vi "Import Configuration and Payload Files.vi"(8 "error in":errorcluster, 9 "payload file path":path, 10 "parameters configuration file path":path, 11 "custom device ref":T1=18446744073709551615 format="%.0x") -> (0 "error out":errorcluster, 3 "custom device ref out":T1=18446744073709551615 format="%.0x")   [LabVIEW 2020, in "AIM ARINC 664 Scripting.lvlib"]
doc: "For the specified <b>custom device ref</b>, imports the parameters configuration file located at the input <b>parameters configuration file path</b>. For successful deployment and operation, the parameters configuration must be consistent with the published schema."
uses:
  AIM ARINC 664 Scripting.lvlib
  <vilib>/NI VeriStand/Custom Device API/Custom Device Item Ref.ctl
  <vilib>/NI VeriStand/Custom Device API/Custom Device API.lvlib
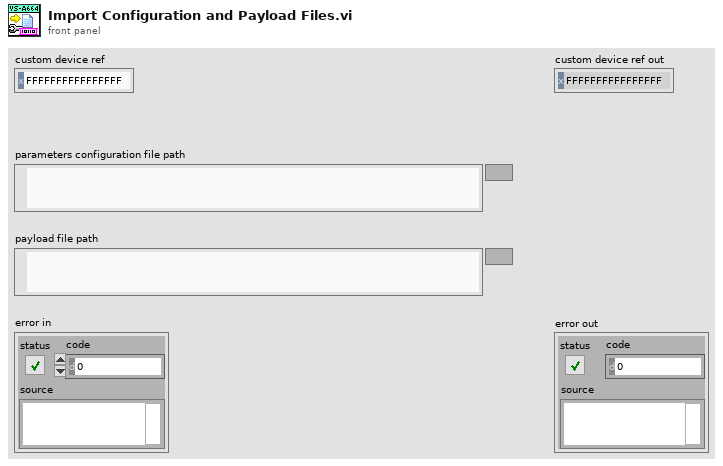
[diagram p1: front panel]
types:
  T1 = typedef "Custom Device API.lvlib/Custom Device Item Ref.ctl" = u64
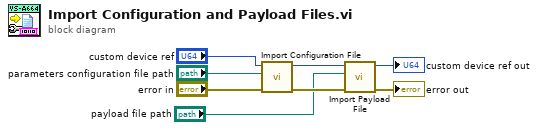
[diagram p0: block diagram]
diagram:
  n1 = call "Import Configuration File.vi"("error in"="error in", "parameters configuration file path"="parameters configuration file path", "custom device ref"="custom device ref") -> ("error out"=w5:errorcluster, "custom device ref out"=w2:T1)  [unwired: 7 in]
  n2 = call "Import Payload File.vi"("error in (no error)"=w5, "payload file path"="payload file path", "custom device ref in"=w2) -> ("error out"=→"error out":errorcluster, "custom device ref out out"=→"custom device ref out":T1)  [unwired: 7 in]
